vi "Destroy.vi"(8 "error in (no error)":errorcluster, 11 "Web FP In":refnum<class "Web Front Panel.lvclass">) -> (0 "error out":errorcluster, 3 "Web FP Out":refnum<class "Web Front Panel.lvclass">)   [LabVIEW 2017, in "Front Panel Publisher.lvlib" / "Web Front Panel.lvclass"]
uses:
  Web Front Panel.lvclass
  Front Panel Objects/Object_class/Object.lvclass
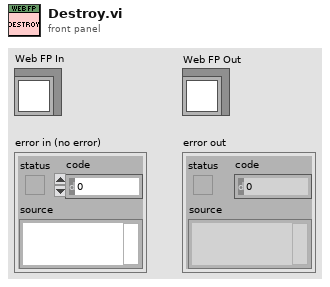
[diagram p1: front panel]
types:
  T1 = typedef "Front Panel Publisher.lvlib/Web Front Panel.lvclass/Object Attributes.ctl" = cluster{"VI Identifier":string, "VI Reference":refnum<vi>, "Controls":refnum<class "Object.lvclass">[], "Indicators":refnum<class "Object.lvclass">[], "Decorations":refnum<class "Object.lvclass">[], "VR With Previous Get":refnum<data-value>, "VR With Ring Images":refnum<data-value>}
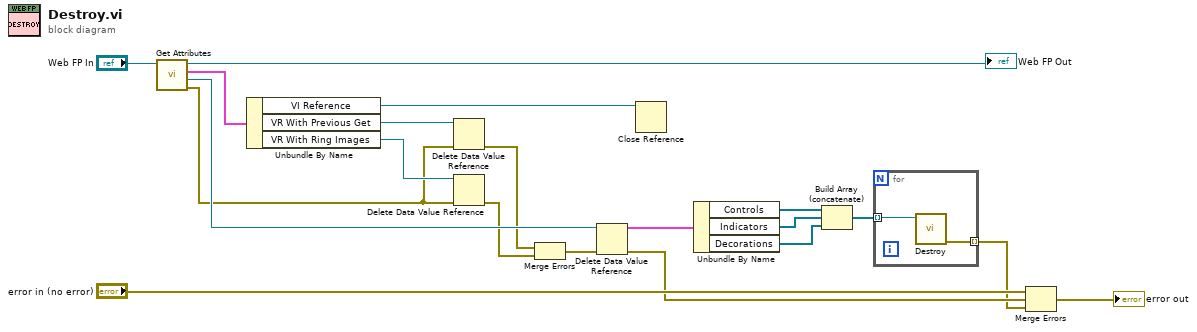
[diagram p0: block diagram]
diagram:
  n1 = call "Get Attributes.vi"("Web FP In"="Web FP In") -> ("error out"=w8:errorcluster, "DataRef"=w17:refnum<data-value>, "Data"=w14:T1, "Web FP Out"=→"Web FP Out":refnum<class "Web Front Panel.lvclass">)  [unwired: 7 in]
  n2 = Unbundle By Name(w14) -> ("VI Reference"=w1:refnum<vi>, "VR With Previous Get"=w13:refnum<data-value>, "VR With Ring Images"=w11:refnum<data-value>)
  n3 = Delete Data Value Reference(data value reference=w13, error in=w8) -> (error out=w12:errorcluster)  [unwired: 1 out]
  n4 = Delete Data Value Reference(data value reference=w11, error in=w8) -> (error out=w9:errorcluster)  [unwired: 1 out]
  n5 = Merge Errors(w12, w9) -> (w10:errorcluster)
  n6 = Delete Data Value Reference(data value reference=w17, error in=w10) -> (data value=w7:T1, error out=w15:errorcluster)
  n7 = Close Reference(reference=w1) -> ()  [unwired: 1 in, 1 out]
  n8 = Unbundle By Name(w7) -> ("Controls"=w6:refnum<class "Object.lvclass">[], "Indicators"=w5:refnum<class "Object.lvclass">[], "Decorations"=w4:refnum<class "Object.lvclass">[])
  n9 = Build Array (concatenate)(w6, w5, w4) -> (w3:refnum<class "Object.lvclass">[])
  n10 = for {
    tunnel: w3 -> [w22] mode=indexing
    tunnel: [w21] -> w2 mode=indexing
    n11 = call-dynamic "Destroy.vi"("Object In"=w22) -> ("error out"=w21:errorcluster)  [unwired: 9 in, 1 out]
  }
  n12 = Merge Errors("error in (no error)", w15, w2) -> (→"error out":errorcluster)
